vi "GA Get Crd Pos.vi"(8 "error in (no error)":errorcluster caption="错误输入（无错误）", 10 "pPos":dbl, 11 "nCrdNum":i16) -> (0 "error out":errorcluster caption="错误输出", 2 "pPos out":dbl, 3 "function return":i32)   [LabVIEW 2015, in "GAS.lvlib"]
doc: "extern \"C\" __declspec(dllimport) int GA_GetCrdPos(short nCrdNum,double *pPos);"
uses:
  <userlib>/BP_GAS/GAS.lvlib
  <userlib>/BP_GAS/GAS.dll
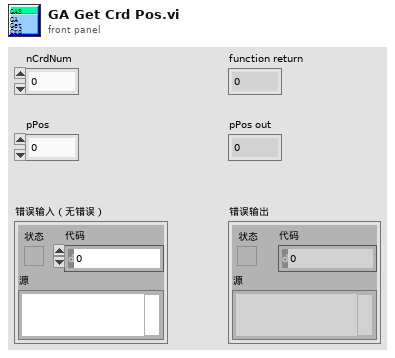
[diagram p1: front panel]
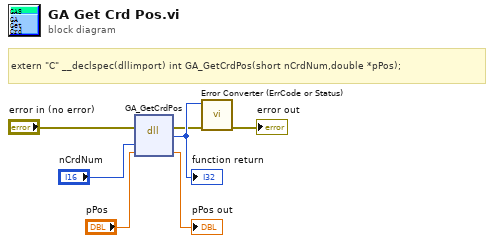
[diagram p0: block diagram]
diagram:
  # "extern \"C\" __declspec(dllimport) int GA_GetCrdPos(short nCrdNum,double *pPos);"
  n1 = dll-call lib="E:/Program Files (x86)/National Instruments/LabVIEW 2015/user.lib/BP_GAS/GAS.*" fn="GA_GetCrdPos"(error in="error in (no error)", "nCrdNum"="nCrdNum", "pPos"="pPos") -> (error out=w2:errorcluster, w7:i32, "pPos"=→"pPos out":dbl)  [unwired: 3 in, 1 out]
  "function return" <- w7
  n2 = call "Error Converter (ErrCode or Status).vi"("error in (no error)"=w2, "error code"=w7) -> ("error out"=→"error out":errorcluster)  [unwired: 9 in]
